vi "SMChart.vi"() -> ()   [LabVIEW 2020]
uses:
  States.ctl
  <vilib>/ErrorRing/Error Ring.xnode
panel:
  in  "stop":bool
  out "Waveform Chart":dbl(graph)
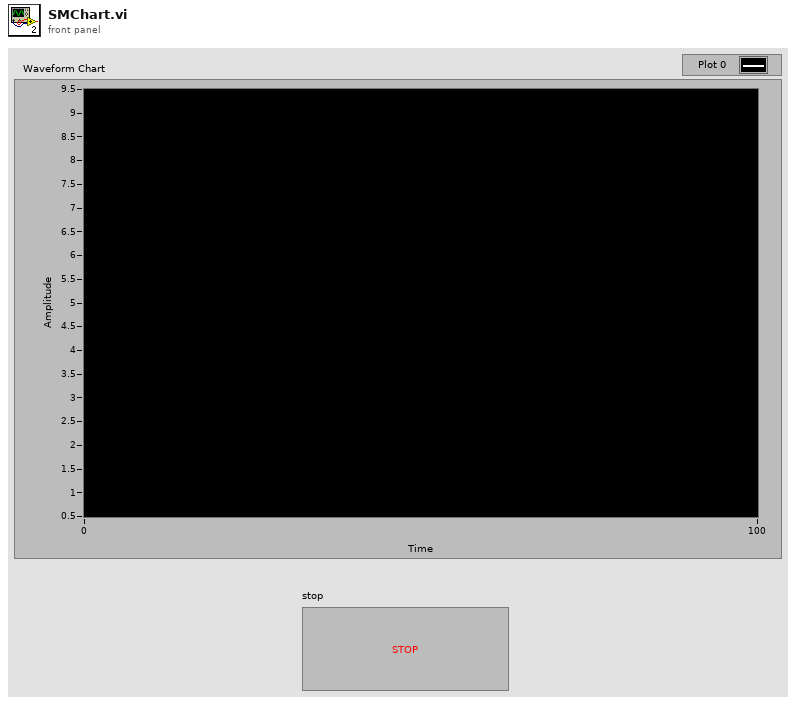
[diagram p1: front panel]
types:
  T1 = typedef "States.ctl" = enum16{"Idle", "DataInit", "UIInit", "RandomNoGen", "UIUpdate", "Exit"}
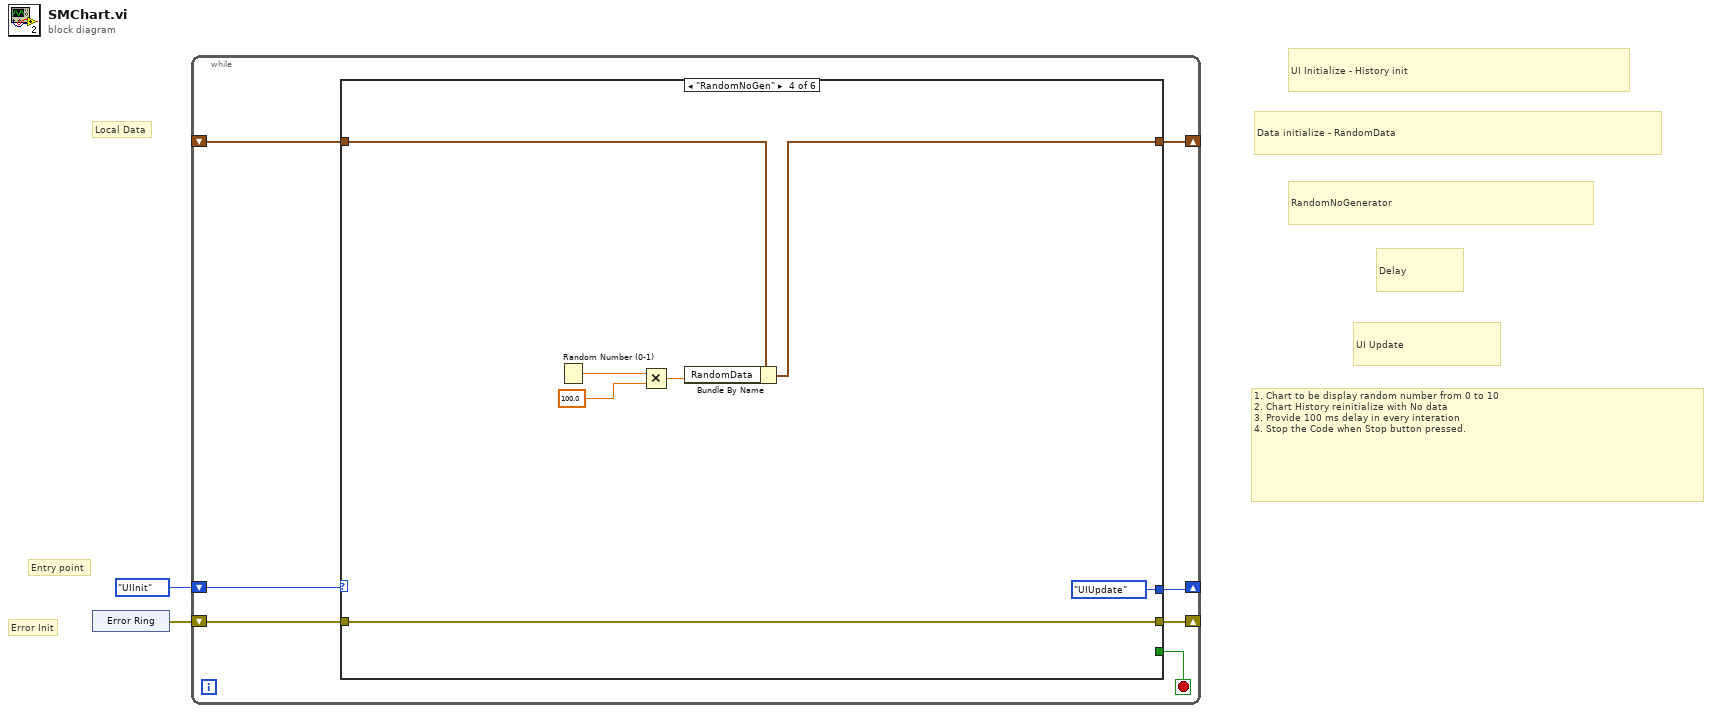
[diagram p0: block diagram]
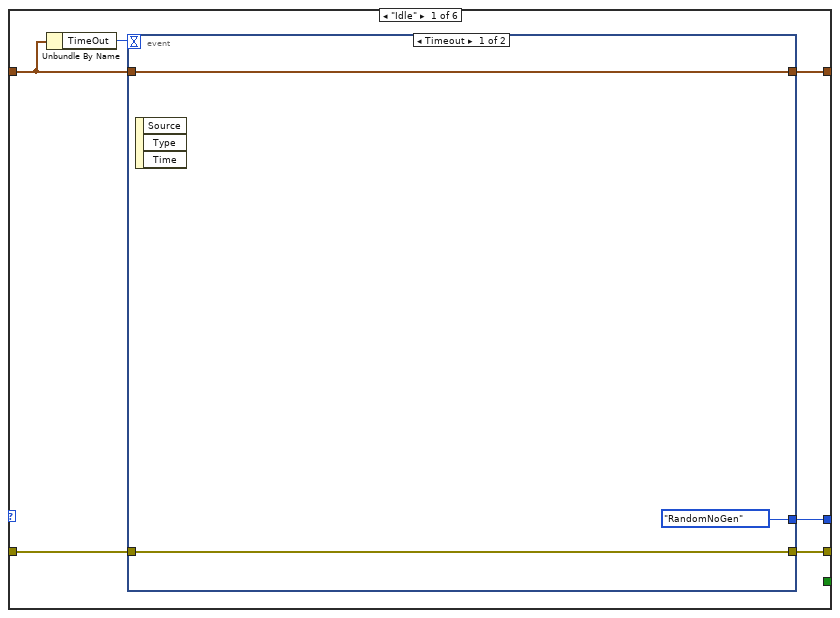
[diagram p2: hidden frame]
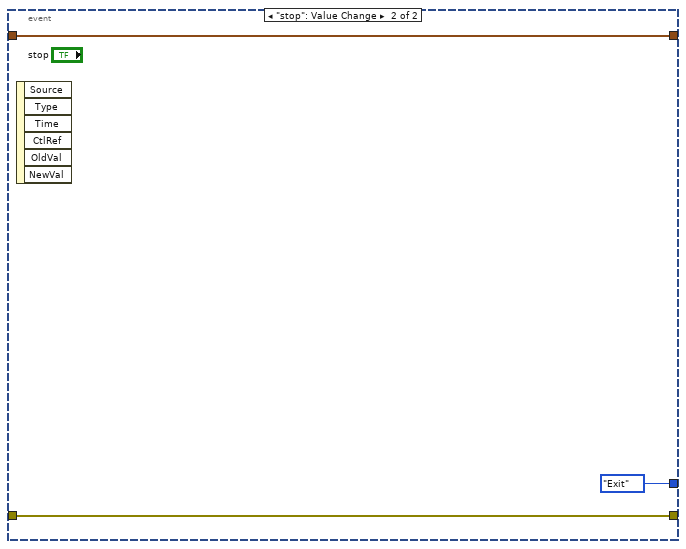
[diagram p3: hidden frame]
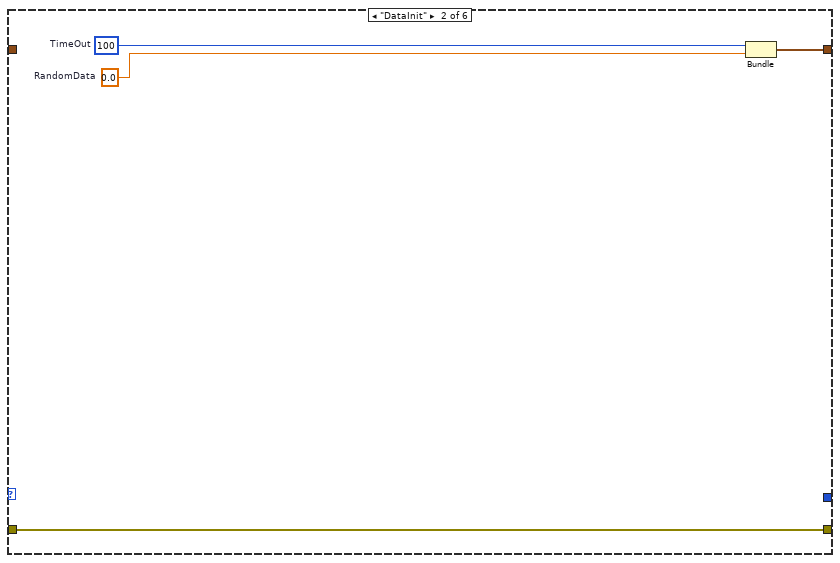
[diagram p4: hidden frame]
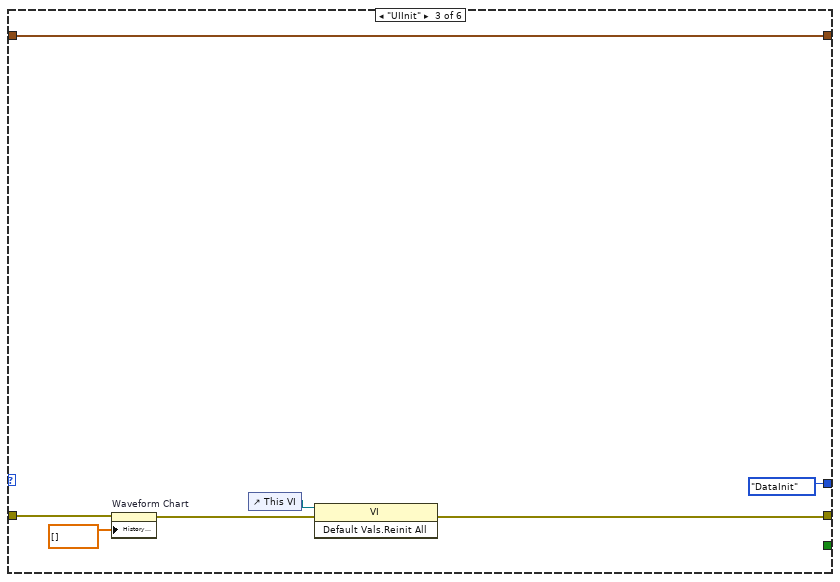
[diagram p5: hidden frame]
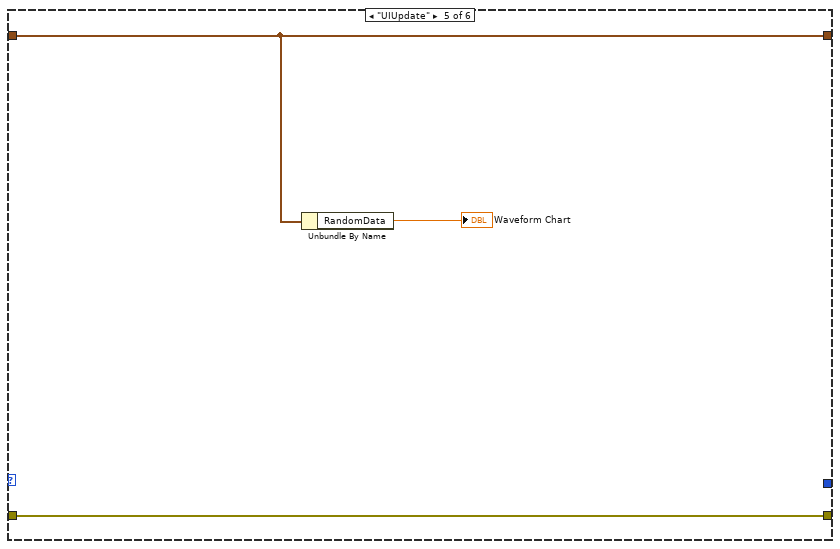
[diagram p6: hidden frame]
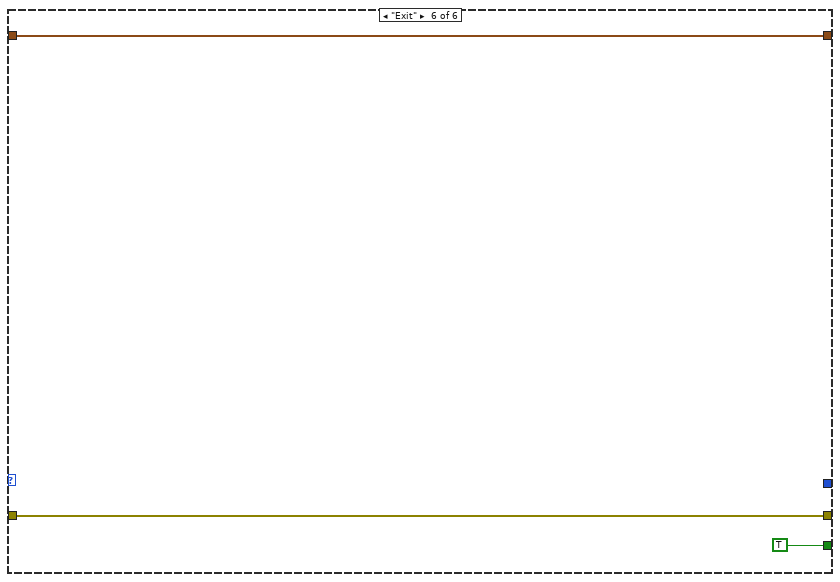
[diagram p7: hidden frame]
diagram:
  # "Local Data"
  # "Error Init"
  # "Entry point"
  # "UI Update"
  # "Delay"
  # "RandomNoGenerator"
  # "Data initialize - RandomData"
  # "UI Initialize - History init"
  # "1. Chart to be display random number from 0 to 10\n2. Chart History reinitialize with No data\n3. Provide 100 ms delay in every interation\n4. Stop the Code when Stop button pressed."
  n1 = xnode "Error Ring"() -> ("error out"=w1:errorcluster)
  n2 = while {
    shift-right: [w4] -> _
    shift-left: States."UIInit" -> [w9]
    shift-right: [w7] -> _
    shift-left: w1 -> [w8]
    shift-right: [w6] -> _
    shift-left: _ -> [w5]
    stop <- w3 stop-if-true
    n3 = case shown="\"RandomNoGen\"" w9 {
      tunnel: w8 -> [w15 w25 w29 w39 w42 w45]
      tunnel: [w14 w25 w27 w39 w42 w45] -> w7
      tunnel: [w13 w24 w32 w38 w41 w44] -> w6
      tunnel: w5 -> [w12 _ w32 w37 w41 w44]
      tunnel: [w10 _ States."DataInit" States."UIUpdate" _ _] -> w4
      tunnel: [_ _ _ _ _ TRUE] -> w3
      frame "Idle" {
        n4 = Unbundle By Name(w12) -> ("TimeOut"=w11:i32)
        n5 = event shown="[0] Timeout" {
          selector: _ -> [_ _]
          dyn-events: _ -> [_ _]
          timeout: w11 -> [_ _]
          tunnel: w15 -> [w18 w21]
          tunnel: [w18 w21] -> w14
          tunnel: w12 -> [w17 w20]
          tunnel: [w17 w20] -> w13
          tunnel: [States."RandomNoGen" States."Exit"] -> w10
          event Timeout {
            n6 = event-data() -> ()  [unwired: 1 in, 3 out]
          }
          event "stop": Value Change {
            n7 = event-data() -> ()  [unwired: 1 in, 6 out]
          }
        }
      }
      frame "DataInit" {
        w22 = 0.0  # RandomData
        w23 = 100  # TimeOut
        n8 = Bundle("TimeOut"=w23, "RandomData"=w22) -> (w24:cluster{"TimeOut":i32, "RandomData":dbl})  [unwired: 1 in]
      }
      frame "UIInit" {
        n9 = property on="Waveform Chart" class="WFChart (strict)"(error in=w29, "History Data"=dbl[] []) -> (error out=w28:errorcluster)  [unwired: 1 in, 1 out]
        n10 = control-ref of="This VI"() -> (w30:refnum<vi>)
        n11 = invoke class="VI" method="Default Vals.Reinit All"(reference=w30, error in=w28) -> (error out=w27:errorcluster)  [unwired: 1 in, 2 out]
      }
      frame "RandomNoGen" {
        n12 = Random Number (0-1)() -> (number: 0 to 1=w36:dbl)
        n13 = Multiply(x=w36, y=100.0) -> (x*y=w34:dbl)
        n14 = Bundle By Name(cluster=w37, "RandomData"=w34) -> (w38:cluster{"TimeOut":i32, "RandomData":dbl})
      }
      frame "UIUpdate" {
        n15 = Unbundle By Name(w41) -> ("RandomData"=→"Waveform Chart":dbl)
      }
      frame "Exit" {
      }
    }
  }
